vi "GEA2 Script_Parse ERD Read.vi"(0 "Data":string, 11 "Error In":errorcluster) -> (2 "Expected Responses":string[](array[string]), 6 "GEA Inputs":T2 {"Destination" format="%.0x"; "Source" format="%.0x"}, 8 "Read ERD List":T1[](array[typedef]) {"ERD Number" format="%.0x"}, 15 "Error Out":errorcluster)   [LabVIEW 2014]
uses:
  type defs/Source_Destination.ctl
  type defs/ERD Read Data In.ctl
  <vilib>/regexp/Match Regular Expression.xnode
  library/GEA2_Toolkit.lvlib
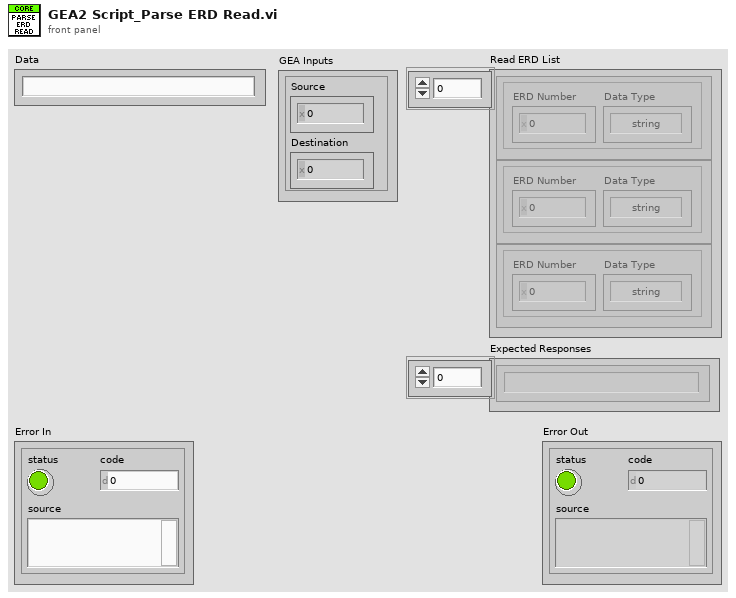
[diagram p1: front panel]
types:
  T1 = typedef "GEA2_Toolkit.lvlib/ERD Read Data In.ctl" = cluster{"ERD Number":u16, "Data Type":enum16{"string", "boolean", "uint8_t", "uint16_t", "uint32_t", "uint64_t"}}
  T2 = typedef "GEA2_Toolkit.lvlib/Source_Destination.ctl" = cluster{"Source":u8, "Destination":u8}
  T3 = enum16{"string", "boolean", "uint8_t", "uint16_t", "uint32_t"}
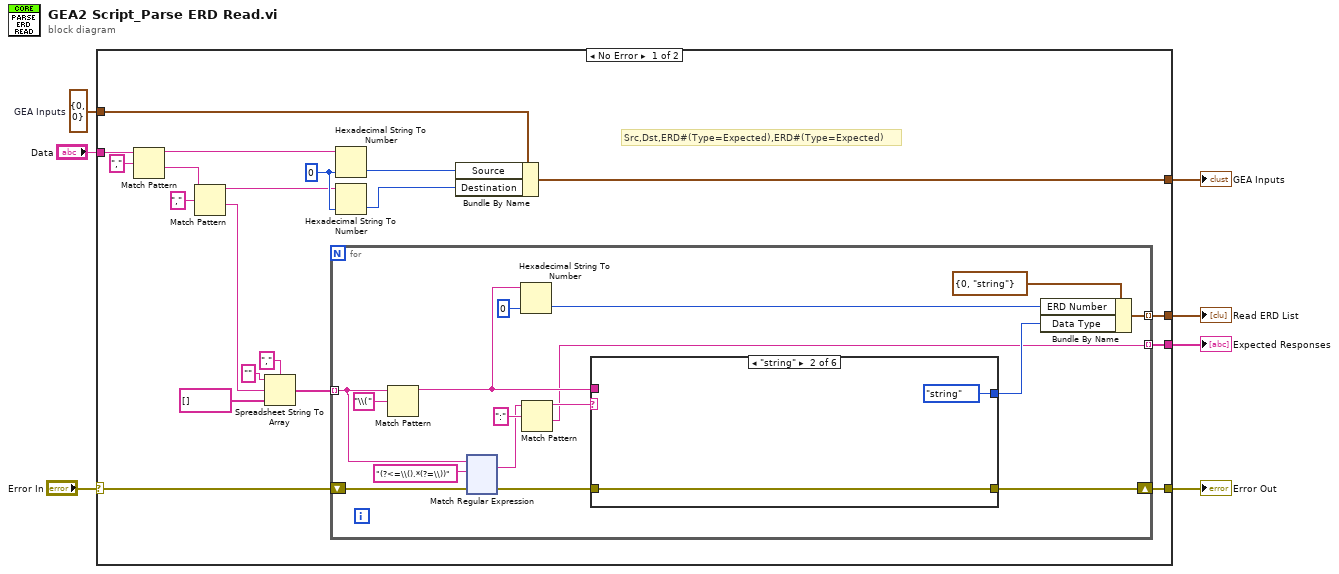
[diagram p0: block diagram]
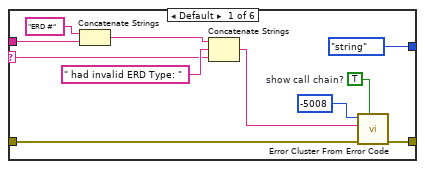
[diagram p2: hidden frame]
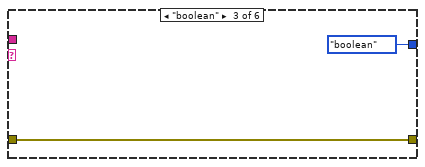
[diagram p3: hidden frame]
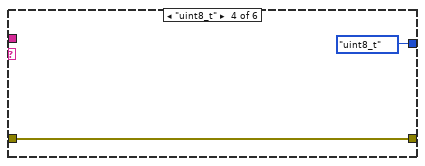
[diagram p4: hidden frame]
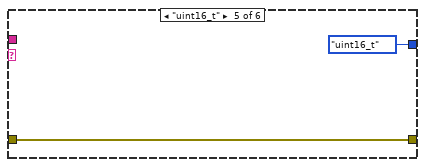
[diagram p5: hidden frame]
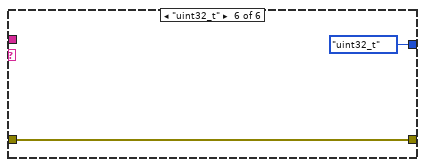
[diagram p6: hidden frame]
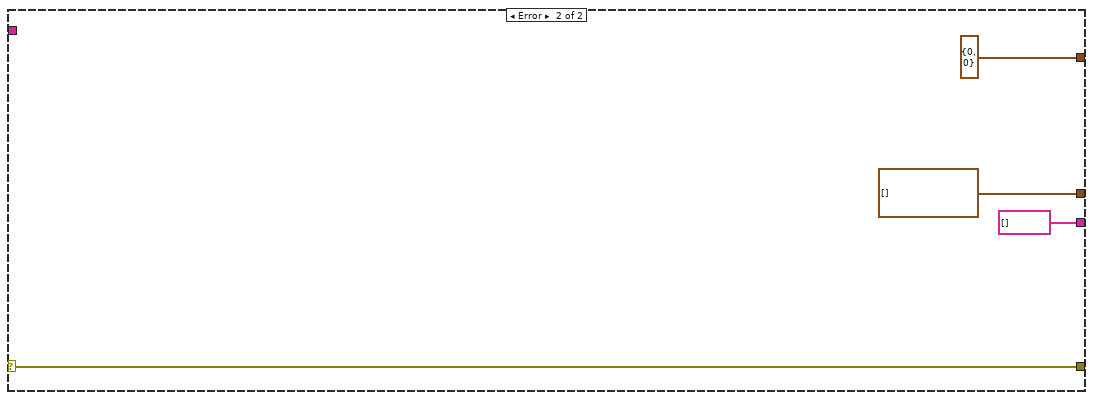
[diagram p7: hidden frame]
diagram:
  w6 = T2 {"Source"=0, "Destination"=0}  # GEA Inputs
  n1 = case shown="No Error" "Error In" {
    selector: "Error In" -> [w16 w182]
    tunnel: "Data" -> [w27 _]
    tunnel: w6 -> [w18 _]
    tunnel: [w17 T2 {"Source"=0, "Destination"=0} ("GEA Inputs")] -> w5
    tunnel: [w15 w182] -> w3
    tunnel: [w9 T1[] []] -> w2
    tunnel: [w8 string[] []] -> w1
    frame No Error {
      w21 = u8 0
      # "Src,Dst,ERD#(Type=Expected),ERD#(Type=Expected)"
      n2 = Match Pattern(string=w27, regular expression=",") -> (before substring=w24:string, after substring=w23:string)  [unwired: 1 in, 2 out]
      n3 = Match Pattern(string=w23, regular expression=",") -> (before substring=w20:string, after substring=w13:string)  [unwired: 1 in, 2 out]
      n4 = Spreadsheet String To Array(delimiter (Tab)=",", format string="", spreadsheet string=w13, array type (2D Dbl)=string[] []) -> (array=w11:string[])
      n5 = for {
        tunnel: [w40] -> w9 mode=indexing
        shift-right: [w37] -> w15
        shift-left: w16 -> [w31]
        tunnel: w11 -> [w30] mode=indexing
        tunnel: [w28] -> w8 mode=indexing
        n6 = Match Pattern(string=w30, regular expression="\\(") -> (before substring=w34:string)  [unwired: 1 in, 3 out]
        n7 = xnode "Match Regular Expression"("input string"=w30, "regular expression"="(?<=\\().*(?=\\))", "error in"=w31) -> ("whole match"=w29:string, "error out"=w32:errorcluster)  [unwired: 3 in, 3 out]
        n8 = Hexadecimal String To Number(string=w34, default (0uL)=u16 0 ("ERD Number")) -> (number=w42:u16)  [unwired: 1 in, 1 out]
        n9 = Match Pattern(string=w29, regular expression=":") -> (before substring=w36:string, after substring=w28:string)  [unwired: 1 in, 2 out]
        n10 = case shown="\"string\"" w36 {
          selector: w36 -> [w162 _ _ _ _ _]
          tunnel: [T3."string" ("Data Type") T3."string" ("Data Type") T3."boolean" ("Data Type") T3."uint8_t" ("Data Type") T3."uint16_t" ("Data Type") T3."uint32_t" ("Data Type")] -> w38
          tunnel: w32 -> [w167 w169 w171 w173 w175 w177]
          tunnel: [w166 w169 w171 w173 w175 w177] -> w37
          tunnel: w34 -> [w159 _ _ _ _ _]
          frame Default {
            w164 = TRUE  # show call chain?
            n11 = Concatenate Strings("ERD #", w159) -> (w158:string)
            n12 = Concatenate Strings(w158, " had invalid ERD Type: " ("error message (\"\")"), w162) -> (w161:string)
            n13 = call <vilib>:"Error Cluster From Error Code.vi"("show call chain? (False)"=w164, "error in (no error)"=w167, "error message (\"\")"=w161, "error code (0)"=-5008) -> ("error out"=w166:errorcluster)  [unwired: 5 in]
          }
          frame "string" {
          }
          frame "boolean" {
          }
          frame "uint8_t" {
          }
          frame "uint16_t" {
          }
          frame "uint32_t" {
          }
        }
        n14 = Bundle By Name(cluster=T1 {"ERD Number"=0, "Data Type"=enum."string"} ("ERD Read Data In"), "ERD Number"=w42, "Data Type"=w38) -> (w40:T1)
      }
      n15 = Hexadecimal String To Number(string=w24, default (0uL)=w21) -> (number=w22:u8)  [unwired: 1 in, 1 out]
      n16 = Hexadecimal String To Number(string=w20, default (0uL)=w21) -> (number=w19:u8)  [unwired: 1 in, 1 out]
      n17 = Bundle By Name(cluster=w18, "Source"=w22, "Destination"=w19) -> (w17:T2)
    }
    frame Error {
    }
  }
  "GEA Inputs" <- w5
  "Error Out" <- w3
  "Read ERD List" <- w2
  "Expected Responses" <- w1
